vi "Resize and Align.vi"(9 "number of channels":i32, 10 "Refnums for Resizing and Alignment":T5, 11 "State in":T1={"Graph Visible Items"={"Plot Legend"=FALSE, "Scale Legend"=FALSE, "Graph Palette"=FALSE, "Cursor Legend"=FALSE, "X Scrollbar"=FALSE}, "View Table"=FALSE, "Table Visible Items"={"Vertical Scrollbar"=FALSE, "Horizontal Scrollbar"=FALSE, "Row Headers"=FALSE, "Column Headers"=FALSE, "Vertical Lines"=FALSE, "Horizontal Lines"=FALSE}, "Header Font"={"Font Name"="", "Size"=0, "Bold"=FALSE, "Italic"=FALSE, "Underline"=FALSE, "Strikeout"=FALSE, "Color"=0}, "Cell Font"={"Font Name"="", "Size"=0, "Bold"=FALSE, "Italic"=FALSE, "Underline"=FALSE, "Strikeout"=FALSE, "Color"=0}, "Description and Tip..."={"Description"="", "Tip"=""}, "Moveable Splitter Position"=0, "Measurement Cursor Configuration"={"XY"={"enable XY"=FALSE, "Position (X)"=[], "Type"=enum."Absolute", "Y reference"=0.0, "color"=0}, "band"={"enable band"=FALSE, "B1"=0.0, "B2"=0.0, "Fixed bandwidth (B2-B1)"=0.0, "B1 color"=0, "B2 color"=0}, "harmonic"={"enable harmonics"=FALSE, "X reference (1X)"=0.0, "Maximum"=0, "Subset"=enum."All", "1X color"=0, "MX color"=0}, "sideband"={"enable sideband"=FALSE, "X center (C)"=0.0, "Sidebands"=0, "X spacing (s)"=0.0, "Center color"=0, "Sideband color"=0}}, "Cursors"={"List"=[], "Tags"=[]}, "X Increment"=0.0, "X Scale"={"Label Visible"=FALSE, "Label Text"="", "Mapping Mode"=0, "Format String"=""}, "Y Scale"={"Label Visible"=FALSE, "Label Text"="", "Mapping Mode"=0, "Format String"=""}, "Colors"={"background"=16777215, "major grid"=8355711, "minor grid"=12632256, "font"=0}, "desired spectrum view"={"scaling"={"linear/dB"=enum."no change", "dB reference"=0.0, "power/magnitude"=enum."no change", "view"=enum."no change"}, "spectral density"=enum."no change"}, "Plot Color Wheel"=[3381759, 32768, 982784, 4375295, 13827953, 13457919, 16757522, 4343295, 16728758, 12095254], "Plots"=[], "registered user events"=variant, "Lock 1X to Peak"=FALSE, "spectrum component"=32, "phase spectrum view"={"desired units"=0, "desired wrapping"=4}} caption="State" {"phase spectrum view"."desired wrapping" items=["No change", "Unwrap", "Wrap: -360 to 0", "Wrap: -270 to 90", "Wrap: -180 to 180", "Wrap: -90 to 270", "Wrap: 0 to 360", "Wrap: custom range"]; "phase spectrum view"."desired units" items=["No change", "Radians", "Degrees", "Cycles"]; "spectrum component" items=["Magnitude^2"=37, "Magnitude"=32, "Phase"=33, "Real"=34, "Imaginary"=35, "Coherence"=36, "Unknown"=99]; "Y Scale"."Mapping Mode" items=["Linear", "Logarithmic", "dB"]; "X Scale"."Mapping Mode" items=["Linear", "Logarithmic"]}) -> (0 "error out":errorcluster, 3 "State out":T1={"Graph Visible Items"={"Plot Legend"=FALSE, "Scale Legend"=FALSE, "Graph Palette"=FALSE, "Cursor Legend"=FALSE, "X Scrollbar"=FALSE}, "View Table"=FALSE, "Table Visible Items"={"Vertical Scrollbar"=FALSE, "Horizontal Scrollbar"=FALSE, "Row Headers"=FALSE, "Column Headers"=FALSE, "Vertical Lines"=FALSE, "Horizontal Lines"=FALSE}, "Header Font"={"Font Name"="", "Size"=0, "Bold"=FALSE, "Italic"=FALSE, "Underline"=FALSE, "Strikeout"=FALSE, "Color"=0}, "Cell Font"={"Font Name"="", "Size"=0, "Bold"=FALSE, "Italic"=FALSE, "Underline"=FALSE, "Strikeout"=FALSE, "Color"=0}, "Description and Tip..."={"Description"="", "Tip"=""}, "Moveable Splitter Position"=0, "Measurement Cursor Configuration"={"XY"={"enable XY"=FALSE, "Position (X)"=[], "Type"=enum."Absolute", "Y reference"=0.0, "color"=0}, "band"={"enable band"=FALSE, "B1"=0.0, "B2"=0.0, "Fixed bandwidth (B2-B1)"=0.0, "B1 color"=0, "B2 color"=0}, "harmonic"={"enable harmonics"=FALSE, "X reference (1X)"=0.0, "Maximum"=0, "Subset"=enum."All", "1X color"=0, "MX color"=0}, "sideband"={"enable sideband"=FALSE, "X center (C)"=0.0, "Sidebands"=0, "X spacing (s)"=0.0, "Center color"=0, "Sideband color"=0}}, "Cursors"={"List"=[], "Tags"=[]}, "X Increment"=0.0, "X Scale"={"Label Visible"=FALSE, "Label Text"="", "Mapping Mode"=0, "Format String"=""}, "Y Scale"={"Label Visible"=FALSE, "Label Text"="", "Mapping Mode"=0, "Format String"=""}, "Colors"={"background"=16777215, "major grid"=8355711, "minor grid"=12632256, "font"=0}, "desired spectrum view"={"scaling"={"linear/dB"=enum."no change", "dB reference"=0.0, "power/magnitude"=enum."no change", "view"=enum."no change"}, "spectral density"=enum."no change"}, "Plot Color Wheel"=[3381759, 32768, 982784, 4375295, 13827953, 13457919, 16757522, 4343295, 16728758, 12095254], "Plots"=[], "registered user events"=variant, "Lock 1X to Peak"=FALSE, "spectrum component"=32, "phase spectrum view"={"desired units"=0, "desired wrapping"=4}} caption="State" {"phase spectrum view"."desired wrapping" items=["No change", "Unwrap", "Wrap: -360 to 0", "Wrap: -270 to 90", "Wrap: -180 to 180", "Wrap: -90 to 270", "Wrap: 0 to 360", "Wrap: custom range"]; "phase spectrum view"."desired units" items=["No change", "Radians", "Degrees", "Cycles"]; "spectrum component" items=["Magnitude^2"=37, "Magnitude"=32, "Phase"=33, "Real"=34, "Imaginary"=35, "Coherence"=36, "Unknown"=99]; "Y Scale"."Mapping Mode" items=["Linear", "Logarithmic", "dB"]; "X Scale"."Mapping Mode" items=["Linear", "Logarithmic"]})   [LabVIEW 2017, in "Spectrum with Cursors.xctl"]
doc: "Based on moveable splitter position and pane sizes, resize the graph and table and align table with plot area."
uses:
  <vilib>/addons/_XControls/Spectrum with Cursors/Spectrum with Cursors.xctl
  <vilib>/addons/_XControls/Spectrum with Cursors/Controls/Refnums Typedef.ctl
  <vilib>/addons/_XControls/Spectrum with Cursors/Controls/State.ctl
  <vilib>/Utility/miscctls.llb/LVFontTypeDef.ctl
  <vilib>/addons/_XControls/Spectrum with Cursors/Controls/Measurement Cursor Configuration.ctl
  <vilib>/addons/_NISVFA/_Shared subVIs/Controls/NI Spectrum Component.ctl
  <vilib>/Utility/miscctls.llb/LVPositionTypeDef.ctl
  <vilib>/Utility/miscctls.llb/LVRowAndColumnTypeDef.ctl
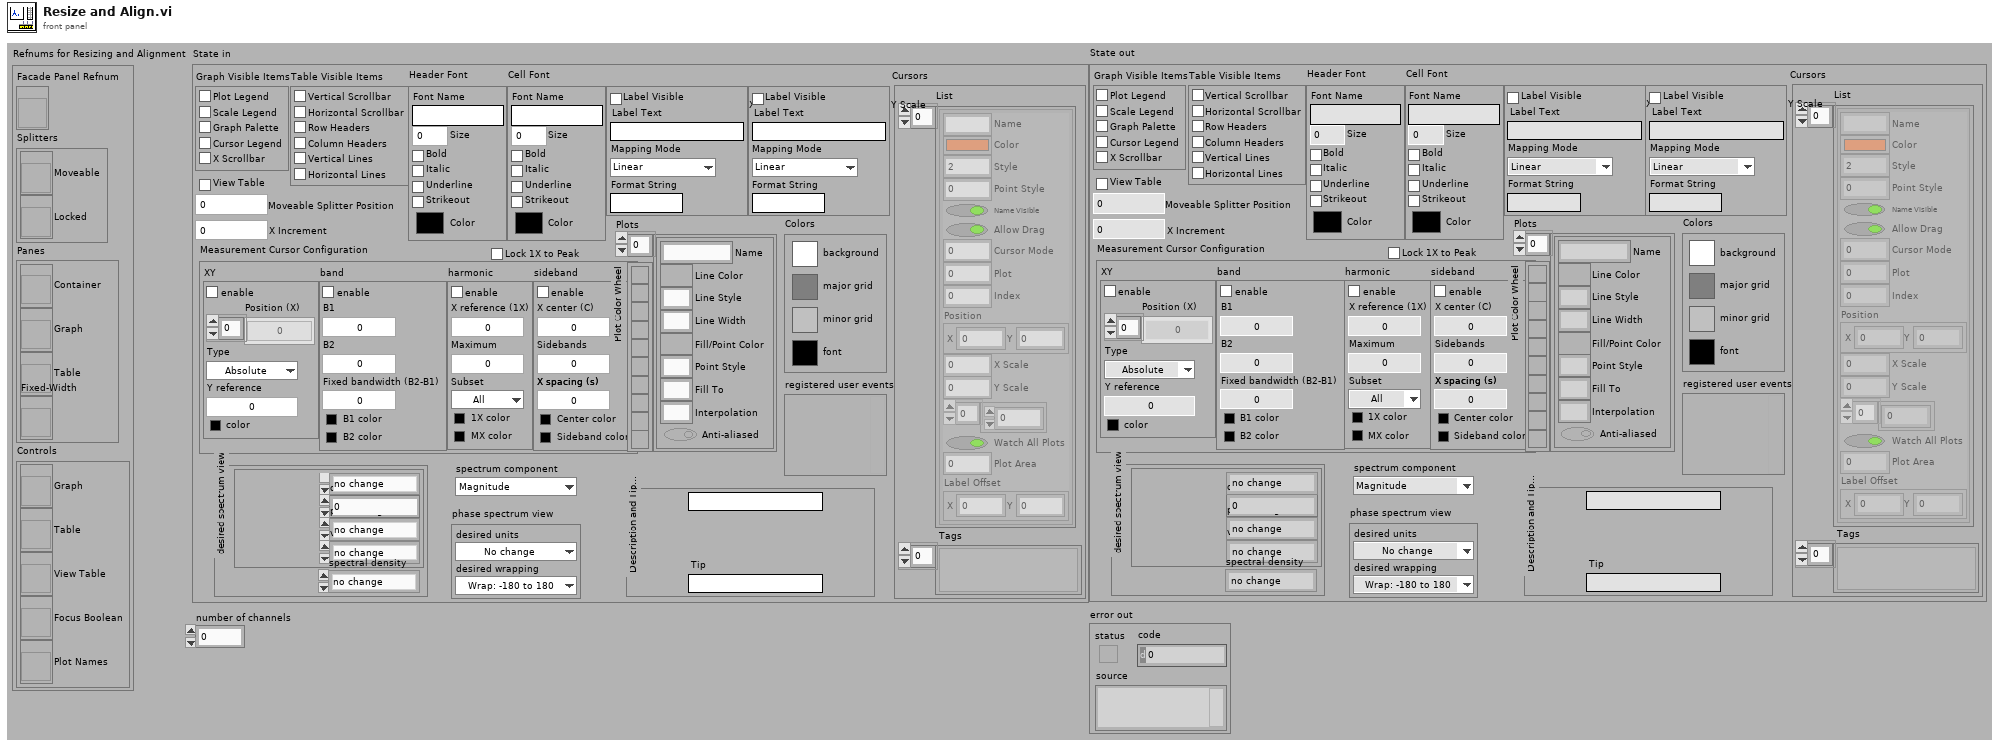
[diagram p1: front panel]
types:
  T1 = typedef "Spectrum with Cursors.xctl/State.ctl" = cluster{"Graph Visible Items":cluster{"Plot Legend":bool, "Scale Legend":bool, "Graph Palette":bool, "Cursor Legend":bool, "X Scrollbar":bool}, "View Table":bool, "Table Visible Items":cluster{"Vertical Scrollbar":bool, "Horizontal Scrollbar":bool, "Row Headers":bool, "Column Headers":bool, "Vertical Lines":bool, "Horizontal Lines":bool}, "Header Font":T2, "Cell Font":T2, "Description and Tip...":cluster{"Description":string, "Tip":string}, "Moveable Splitter Position":i32, "Measurement Cursor Configuration":T3, "Cursors":cluster{"List":cluster{"Name":string, "Color":u32, "Style":i32, "Point Style":u8, "Name Visible":bool, "Allow Drag":bool, "Cursor Mode":u32, "Plot":i32, "Index":i32, "Position":cluster{"X":dbl, "Y":dbl}, "X Scale":u32, "Y Scale":u32, "Watch Plots":i32[], "Watch All Plots":bool, "Plot Area":i32, "Label Offset":cluster{"X":dbl, "Y":dbl}}[], "Tags":variant[]}, "X Increment":dbl, "X Scale":cluster{"Label Visible":bool, "Label Text":string, "Mapping Mode":u8, "Format String":string}, "Y Scale":cluster{"Label Visible":bool, "Label Text":string, "Mapping Mode":u8, "Format String":string}, "Colors":cluster{"background":u32, "major grid":u32, "minor grid":u32, "font":u32}, "desired spectrum view":cluster{"scaling":cluster{"linear/dB":enum16{"no change", "linear", "dB"}, "dB reference":dbl, "power/magnitude":enum16{"no change", "power", "magnitude"}, "view":enum16{"no change", "rms", "peak", "peak-peak"}}, "spectral density":enum16{"no change", "spectrum", "spectral density"}}, "Plot Color Wheel":u32[], "Plots":cluster{"Name":string, "Line Color":u32, "Line Style":u8, "Line Width":u8, "Fill/Point Color":u32, "Point Style":u8, "Fill To":i16, "Interpolation":u8, "Anti-aliased":bool}[], "registered user events":variant, "Lock 1X to Peak":bool, "spectrum component":T4, "phase spectrum view":cluster{"desired units":u16, "desired wrapping":u16}}
  T2 = typedef "LVFontTypeDef.ctl" = cluster{"Font Name":string, "Size":u16, "Bold":bool, "Italic":bool, "Underline":bool, "Strikeout":bool, "Color":u32}
  T3 = typedef "Spectrum with Cursors.xctl/Measurement Cursor Configuration.ctl" = cluster{"XY":cluster{"enable XY":bool, "Position (X)":dbl[], "Type":enum16{"Absolute", "Relative"}, "Y reference":dbl, "color":u32}, "band":cluster{"enable band":bool, "B1":dbl, "B2":dbl, "Fixed bandwidth (B2-B1)":dbl, "B1 color":u32, "B2 color":u32}, "harmonic":cluster{"enable harmonics":bool, "X reference (1X)":dbl, "Maximum":i32, "Subset":enum16{"All", "Even", "Odd"}, "1X color":u32, "MX color":u32}, "sideband":cluster{"enable sideband":bool, "X center (C)":dbl, "Sidebands":i32, "X spacing (s)":dbl, "Center color":u32, "Sideband color":u32}}
  T4 = typedef "NI Spectrum Component.ctl" = u16
  T5 = typedef "Spectrum with Cursors.xctl/Refnums Typedef.ctl" = cluster{"Facade Panel Refnum":refnum<vi>, "Splitters":cluster{"Moveable":refnum<vi>, "Locked":refnum<vi>}, "Panes":cluster{"Container":refnum<vi>, "Graph":refnum<vi>, "Table":refnum<vi>, "Fixed-Width":refnum<vi>}, "Controls":cluster{"Graph":refnum<vi>, "Table":refnum<vi>, "View Table":refnum<vi>, "Focus Boolean":refnum<vi>, "Plot Names":refnum<vi>}}
  T6 = typedef "LVPositionTypeDef.ctl" = cluster{"Left":i32, "Top":i32}
  T7 = typedef "LVRectTypeDef.ctl" = cluster{"Left":i16, "Top":i16, "Right":i16, "Bottom":i16}
  T8 = typedef "LVRowAndColumnTypeDef.ctl" = cluster{"Row":i32, "Column":i32}
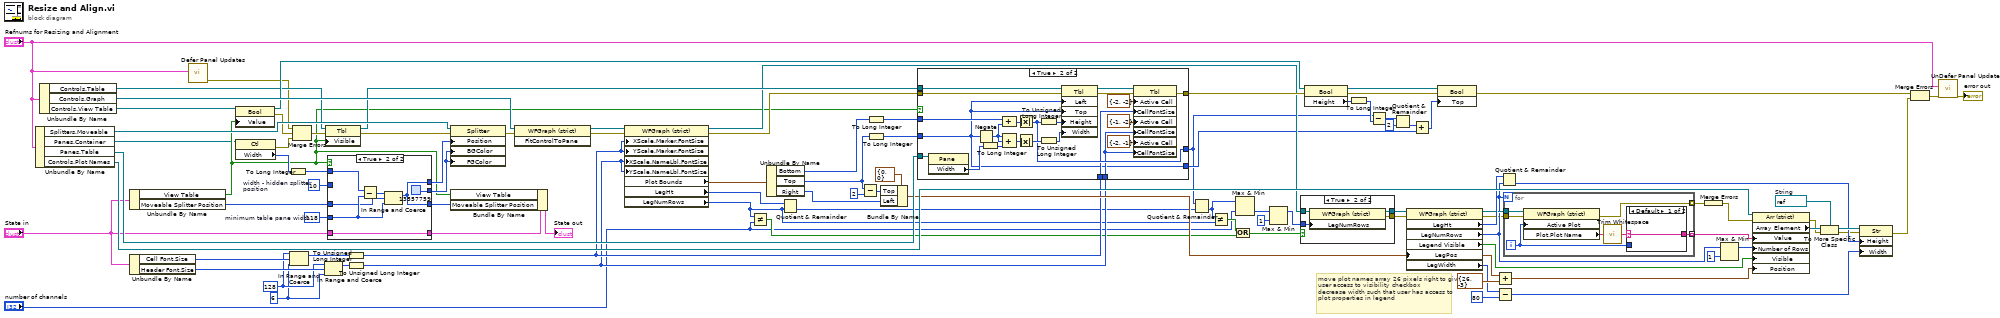
[diagram p0: block diagram]
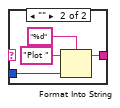
[diagram p3: hidden frame]
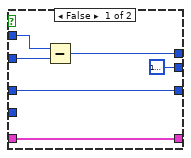
[diagram p4: hidden frame]
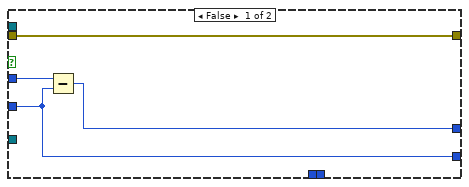
[diagram p5: hidden frame]
diagram:
  w53 = u16 128 ("upper limit")
  w52 = u16 6 ("lower limit")
  w72 = refnum<vi> refnum  # String
  w73 = 118  # minimum table pane width
  w8 = 10  # width - hidden splitter position
  # "move plot names array 26 pixels right to give user access to visibility checkbox\ndecrease width such that user has access to plot properties in legend"
  n1 = Unbundle By Name("Refnums for Resizing and Alignment") -> ("Splitters.Moveable"=w93:refnum<vi>, "Panes.Container"=w6:refnum<vi>, "Panes.Table"=w89:refnum<vi>, "Controls.Plot Names"=w58:refnum<vi>)
  n2 = Unbundle By Name("Refnums for Resizing and Alignment") -> ("Controls.Table"=w17:refnum<vi>, "Controls.Graph"=w95:refnum<vi>, "Controls.View Table"=w18:refnum<vi>)
  n3 = Unbundle By Name("State in") -> ("View Table"=w7:bool, "Moveable Splitter Position"=w87:i32)
  n4 = Unbundle By Name("State in") -> ("Cell Font.Size"=w54:u16, "Header Font.Size"=w55:u16)
  n5 = call <vilib>:"Defer Panel Updates.vi"("Refnums for FP Objects"="Refnums for Resizing and Alignment") -> ("error out"=w4:errorcluster)  [unwired: 9 in, 1 out]
  n6 = property class="Bool"(reference=w18, "Value"=w7) -> (reference out=w86:refnum<vi>, error out=w9:errorcluster)  [unwired: 1 in]
  n7 = property class="Ctl"(reference=w6) -> (error out=w94:errorcluster, "Width"=w92:u32)  [unwired: 1 in, 1 out]
  n8 = To Long Integer(number=w92) -> (32bit integer=w75:i32)
  n9 = In Range and Coerce(upper limit=w53, x=w54, lower limit=w52) -> (coerced(x)=w49:u16)  [unwired: 1 out]
  n10 = Merge Errors(w4, w9, w94) -> (w12:errorcluster)
  n11 = In Range and Coerce(upper limit=w53, x=w55, lower limit=w52) -> (coerced(x)=w48:u16)  [unwired: 1 out]
  n12 = property class="Tbl"(reference=w17, error in=w12, "Visible"=w7) -> (reference out=w50:refnum<vi>, error out=w51:errorcluster)
  n13 = case shown="True" w7 {
    tunnel: w75 -> [w102 w110]
    tunnel: [w100 w111] -> w91
    tunnel: [u32 16777216 ("Color Box") u32 13557759 ("Color Box")] -> w90
    tunnel: [w104 w111] -> w74
    tunnel: w87 -> [w104 w106]
    tunnel: w73 -> [_ w109]
    tunnel: "State in" -> [w103 w108]
    tunnel: [w103 w108] -> w11
    tunnel: w8 -> [w101 _]
    frame False {
      n14 = Subtract(x=w102, y=w101) -> (x-y=w100:i32)
    }
    frame True {
      n15 = Subtract(x=w110, y=w109) -> (x-y=w112:i32)
      n16 = In Range and Coerce(upper limit=w112, x=w106, lower limit=w109) -> (coerced(x)=w111:i32)  [unwired: 1 out]
    }
  }
  n17 = To Unsigned Long Integer(number=w49) -> (unsigned 32bit integer=w47:u32)
  n18 = To Unsigned Long Integer(number=w48) -> (unsigned 32bit integer=w46:u32)
  n19 = property class="Splitter"(reference=w93, error in=w51, "Position"=w91, "BGColor"=w90, "FGColor"=w90) -> (error out=w97:errorcluster)  [unwired: 1 out]
  n20 = Bundle By Name(cluster=w11, "View Table"=w7, "Moveable Splitter Position"=w74) -> (→"State out":T1)
  n21 = invoke class="WFGraph (strict)" method="FitControlToPane"(reference=w95, error in=w97) -> (reference out=w99:refnum<vi>, error out=w98:errorcluster)  [unwired: 1 in, 1 out]
  n22 = property class="WFGraph (strict)"(reference=w99, error in=w98, "XScale.Marker.FontSize"=w47, "YScale.Marker.FontSize"=w47, "XScale.NameLbl.FontSize"=w46, "YScale.NameLbl.FontSize"=w46) -> (reference out=w34:refnum<vi>, error out=w96:errorcluster, "Plot Bounds"=w42:T7, "LegHt"=w24:u32, "LegNumRows"=w20:u32)
  n23 = Not Equal?(x=w20, y="number of channels") -> (x != y?=w25:bool)
  n24 = Unbundle By Name(w42) -> ("Bottom"=w41:i16, "Top"=w64:i16, "Right"=w65:i16)
  n25 = Quotient & Remainder(x=w24, y=w20) -> (floor(x/y)=w22:u32)  [unwired: 1 out]
  n26 = Subtract(x=w64, y=i16 2) -> (x-y=w63:i16)
  n27 = To Long Integer(number=w41) -> (32bit integer=w76:i32)
  n28 = To Long Integer(number=w64) -> (32bit integer=w45:i32)
  n29 = Bundle By Name(cluster=T6 {"Left"=0, "Top"=0} ("Legend:Position"), "Top"=w63, "Left"=w65) -> (w56:T6)
  n30 = case shown="True" w7 {
    tunnel: w50 -> [_ w138]
    tunnel: w45 -> [w113 w117]
    tunnel: w76 -> [w115 w137]
    tunnel: w89 -> [_ w135]
    tunnel: w96 -> [w116 w132]
    tunnel: [w116 w118] -> w83
    tunnel: [w114 w124] -> w21
    tunnel: w47 -> [_ w122]
    tunnel: w46 -> [_ w119]
    tunnel: [w113 w117] -> w23
    frame False {
      n31 = Subtract(x=w115, y=w113) -> (x-y=w114:i32)
    }
    frame True {
      n32 = property class="Pane"(reference=w135) -> ("Width"=w134:u32)  [unwired: 1 in, 2 out]
      n33 = Negate(x=w117) -> (-x=w129:i32)
      n34 = To Long Integer(number=w134) -> (32bit integer=w130:i32)
      n35 = Compound Arithmetic op=ADD(w137, w129) -> (w136:i32)
      n36 = Compound Arithmetic op=ADD(w129, w129, w130) -> (w133:i32)
      n37 = Absolute Value(x=w136) -> (abs(x)=w124:i32)
      n38 = Absolute Value(x=w133) -> (abs(x)=w127:i32)
      n39 = To Unsigned Long Integer(number=w124) -> (unsigned 32bit integer=w131:u32)
      n40 = To Unsigned Long Integer(number=w127) -> (unsigned 32bit integer=w128:u32)
      n41 = property class="Tbl"(reference=w138, error in=w132, "Left"=w117, "Top"=w117, "Height"=w131, "Width"=w128) -> (reference out=w126:refnum<vi>, error out=w125:errorcluster)
      n42 = property class="Tbl"(reference=w126, error in=w125, "Active Cell"=T8 {"Row"=-2, "Column"=-2} ("Active Cell:Active Cell"), "CellFontSize"=w122, "Active Cell"=T8 {"Row"=-1, "Column"=-2} ("Active Cell:Active Cell"), "CellFontSize"=w119, "Active Cell"=T8 {"Row"=-2, "Column"=-1} ("Active Cell:Active Cell"), "CellFontSize"=w119) -> (error out=w118:errorcluster)  [unwired: 1 out]
    }
  }
  n43 = Quotient & Remainder(x=w21, y=w22) -> (floor(x/y)=w14:u32)  [unwired: 1 out]
  n44 = Not Equal?(x=w14, y=w20) -> (x != y?=w19:bool)
  n45 = Or(x=w19, y=w25) -> (x .or. y?=w26:bool)
  n46 = Max & Min(x=w14, y="number of channels") -> (min(x,y)=w15:u32)  [unwired: 1 out]
  n47 = Max & Min(x=w15, y=u32 1 ("lower limit")) -> (max(x,y)=w13:u32)  [unwired: 1 out]
  n48 = case shown="True" w26 {
    tunnel: w34 -> [w139 w143]
    tunnel: [w139 w142] -> w33
    tunnel: w13 -> [_ w141]
    tunnel: [_ w140] -> w32
    frame False {
    }
    frame True {
      n49 = property on="Property Node" class="WFGraph (strict)"(reference=w143, "LegNumRows"=w141) -> (reference out=w142:refnum<vi>, error out=w140:errorcluster)  [unwired: 1 in]
    }
  }
  n50 = property class="Bool"(reference=w86, error in=w83) -> (reference out=w85:refnum<vi>, error out=w82:errorcluster, "Height"=w84:u32)
  n51 = To Long Integer(number=w84) -> (32bit integer=w81:i32)
  n52 = Subtract(x=w21, y=w81) -> (x-y=w80:i32)
  n53 = Quotient & Remainder(x=w80, y=2) -> (floor(x/y)=w78:i32)  [unwired: 1 out]
  n54 = property on="Property Node" class="WFGraph (strict)"(reference=w33, error in=w32, "LegPos"=w56) -> (reference out=w39:refnum<vi>, error out=w31:errorcluster, "LegHt"=w43:u32, "LegNumRows"=w35:u32, "Legend Visible"=w44:bool, "LegWidth"=w57:u32)
  n55 = Add(x=w78, y=w23) -> (x+y=w77:i32)
  n56 = property class="Bool"(reference=w85, error in=w82, "Top"=w77) -> (error out=w37:errorcluster)  [unwired: 1 out]
  n57 = Add(x=w56, y=T6 {"Left"=26, "Top"=-3}) -> (x+y=w68:T6)
  n58 = Subtract(x=w57, y=u32 80) -> (x-y=w59:u32)
  n59 = Quotient & Remainder(x=w43, y=w35) -> (floor(x/y)=w62:u32)  [unwired: 1 out]
  n60 = for {
    N: w35 -> [_]
    tunnel: [w150] -> w60 mode=indexing
    tunnel: w39 -> [w149]
    tunnel: w31 -> [w145]
    tunnel: [w144] -> w30 mode=indexing
    i -> [w146]
    n61 = property on="Property Node" class="WFGraph (strict)"(reference=w149, error in=w145, "Active Plot"=w146) -> (error out=w144:errorcluster, "Plot.Plot Name"=w148:string)  [unwired: 1 out]
    n62 = call <vilib>:"Trim Whitespace.vi"("string"=w148) -> ("trimmed string"=w147:string)  [unwired: 1 in]
    n63 = case shown="Default" w147 {
      selector: w147 -> [w151 _]
      tunnel: w146 -> [_ w155]
      tunnel: [w151 w152] -> w150
      frame Default {
      }
      frame "" {
        n64 = Format Into String(format string="%d", initial string="Plot ", w155) -> (resulting string=w152:string)  [unwired: 1 in, 1 out]
      }
    }
  }
  n65 = Merge Errors(w30) -> (w29:errorcluster)
  n66 = Max & Min(x=w35, y=u32 1 ("lower limit")) -> (max(x,y)=w38:u32)  [unwired: 1 out]
  n67 = property on="Property Node" class="Arr (strict)"(reference=w58, error in=w29, "Value"=w60, "Number of Rows"=w38, "Visible"=w44, "Position"=w68) -> (error out=w28:errorcluster, "Array Element"=w61:refnum<vi>)  [unwired: 1 out]
  n68 = To More Specific Class(target class=w72, reference=w61, error in=w28) -> (specific class reference=w71:refnum<vi>, error out=w27:errorcluster)
  n69 = property class="Str"(reference=w71, error in=w27, "Height"=w62, "Width"=w59) -> (error out=w36:errorcluster)  [unwired: 1 out]
  n70 = Merge Errors(w37, w36) -> (w5:errorcluster)
  n71 = call <vilib>:"UnDefer Panel Updates.vi"("error in (no error)"=w5, "Refnums for FP Objects"="Refnums for Resizing and Alignment") -> ("error out"=→"error out":errorcluster)  [unwired: 8 in, 1 out]
